vi "lvstyx_connect.vi"(2 "error in (no error)":errorcluster, 3 "connection ptr":u32) -> (0 "error out":errorcluster, 1 "client ptr":u32 format="%08x")   [LabVIEW 2010, in "lib1299.lvlib"]
uses:
  lib1299.lvlib
  cstyx/win32/cstyx.dll
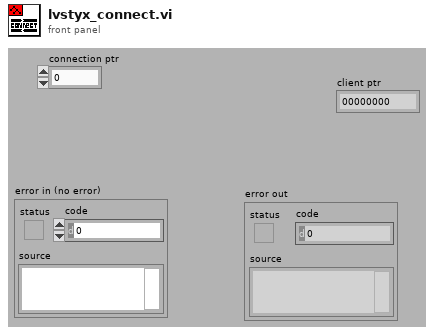
[diagram p1: front panel]
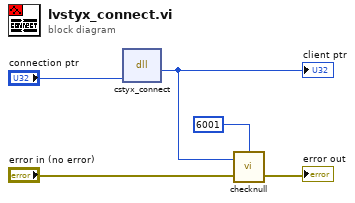
[diagram p0: block diagram]
diagram:
  n1 = dll-call lib="C:/work/ads1299evm/lib_1299/Styx/cstyx/win32/cstyx.dll" fn="cstyx_connect"("connection"="connection ptr") -> (w5:u32)  [unwired: 4 in, 2 out]
  "client ptr" <- w5
  n2 = call "checknull.vi"("error in (no error)"="error in (no error)", "ptr"=w5, "error code"=6001) -> ("error out"=→"error out":errorcluster)  [unwired: 2 in]
